vi "GrabImageDisplay.vi"(2 "error in (no error)":errorcluster, 3 "Image Src":T1, 4 "IBaseData":refnum<k24>) -> (0 "error out":errorcluster, 1 "Image out":T1)   [LabVIEW 2013, in "GxLVlib.lvlib"]
uses:
  GxLVlib.lvlib
  C:/Program Files/Daheng Imaging/GalaxySDK/Samples/LabVIEW SDK/x64/GxLVLib/dll/GxIAPINET.dll
  dll/GxIAPINET.dll
  <vilib>/vision/Image Controls.llb/IMAQ Image.ctl
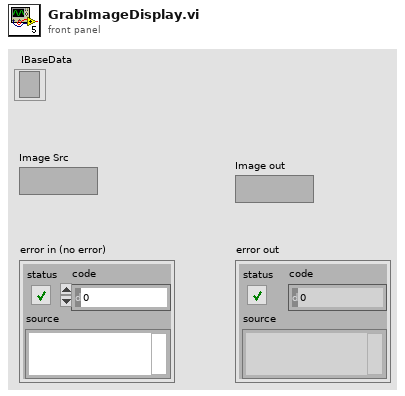
[diagram p1: front panel]
types:
  T1 = typedef "IMAQ Image.ctl" = refnum<image>
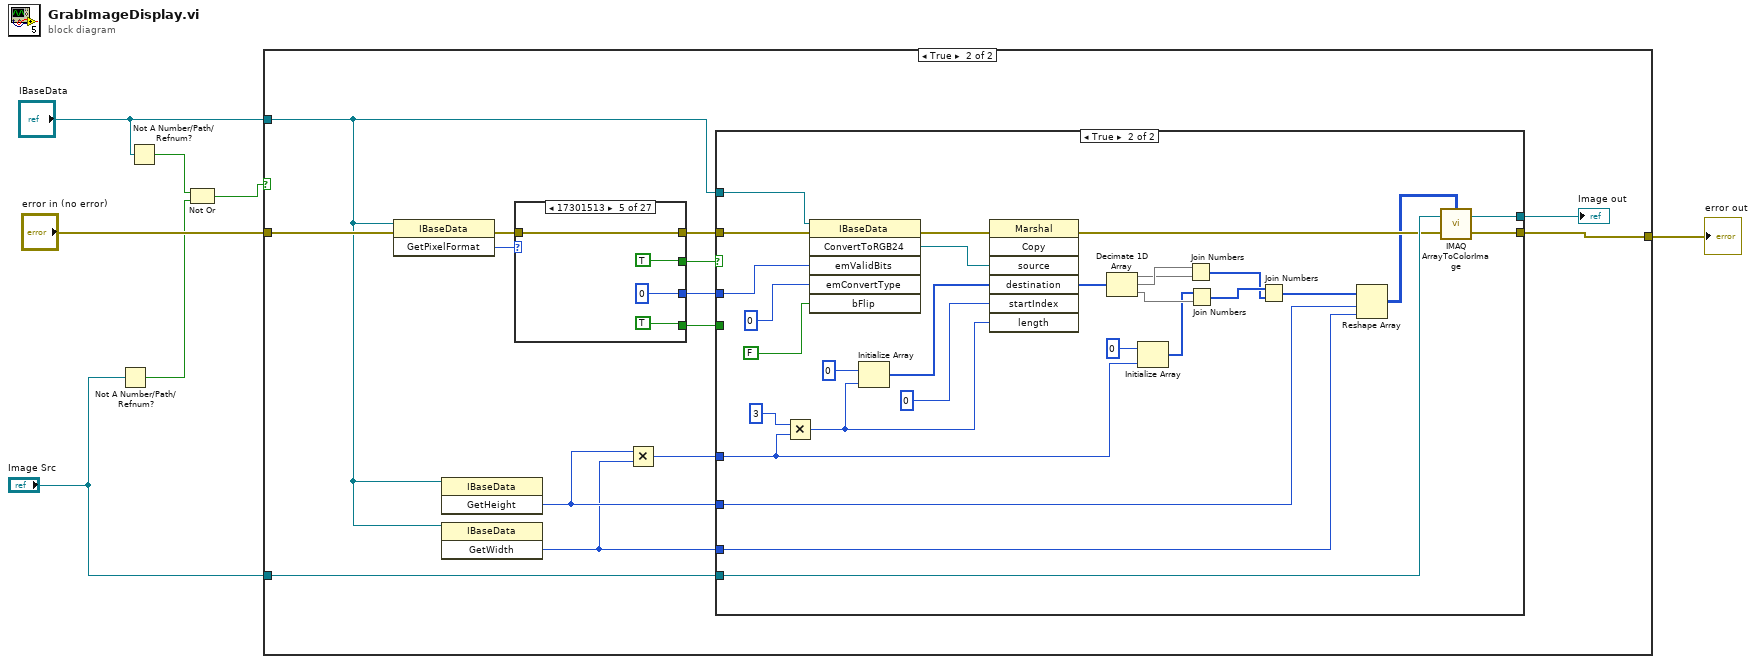
[diagram p0: block diagram]
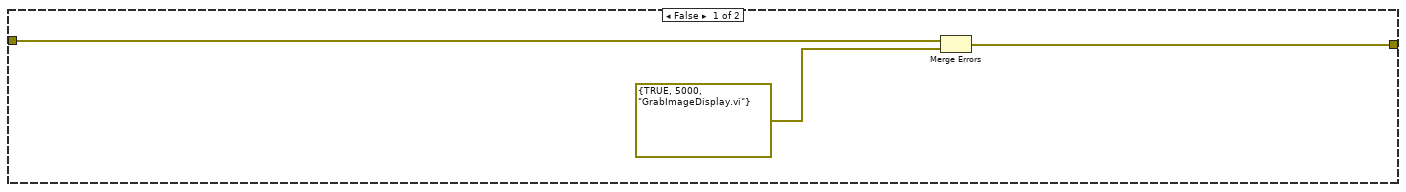
[diagram p2: hidden frame]
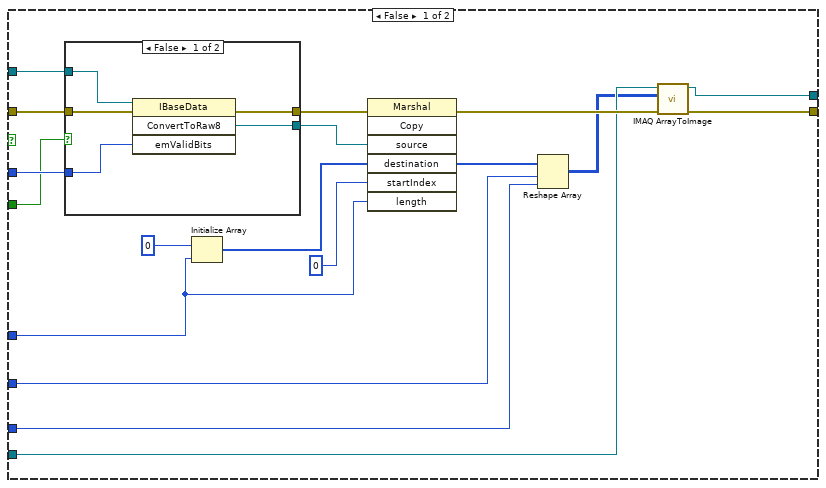
[diagram p3: hidden frame]
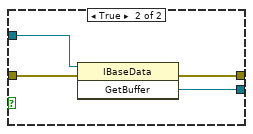
[diagram p4: hidden frame]
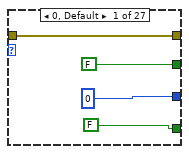
[diagram p5: hidden frame]
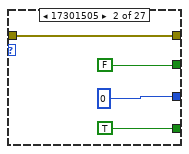
[diagram p6: hidden frame]
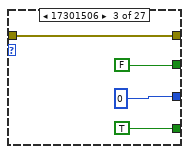
[diagram p7: hidden frame]
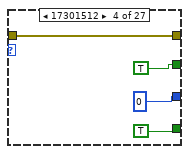
[diagram p8: hidden frame]
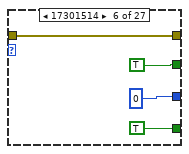
[diagram p9: hidden frame]
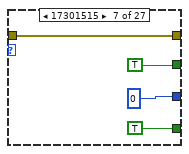
[diagram p10: hidden frame]
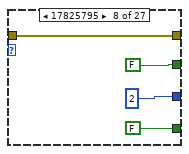
[diagram p11: hidden frame]
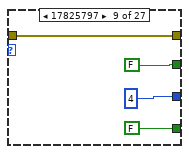
[diagram p12: hidden frame]
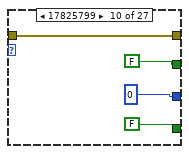
[diagram p13: hidden frame]
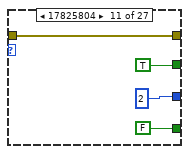
[diagram p14: hidden frame]
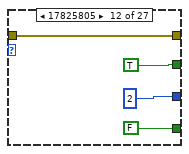
[diagram p15: hidden frame]
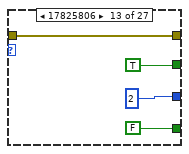
[diagram p16: hidden frame]
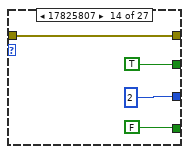
[diagram p17: hidden frame]
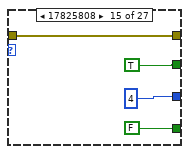
[diagram p18: hidden frame]
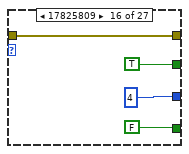
[diagram p19: hidden frame]
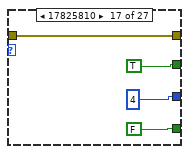
[diagram p20: hidden frame]
diagram:
  n1 = Not A Number/Path/Refnum?(number/path/refnum="Image Src") -> (NaN/Path/Refnum?=w3:bool)
  n2 = Not A Number/Path/Refnum?(number/path/refnum="IBaseData") -> (NaN/Path/Refnum?=w2:bool)
  n3 = Not Or(1:w3, 2:w2) -> (0:w1:bool)
  n4 = case shown="True" w1 {
    tunnel: "IBaseData" -> [_ w14]
    tunnel: "error in (no error)" -> [w10 w22]
    tunnel: [w8 w16] -> w5
    tunnel: "Image Src" -> [_ w17]
    frame False {
      n5 = Merge Errors(w10, errorcluster {TRUE, 5000, "GrabImageDisplay.vi"}) -> (w8:errorcluster)
    }
    frame True {
      n6 = invoke class="IBaseData" method="GetPixelFormat"(reference=w14, error in=w22) -> (error out=w19:errorcluster, "GetPixelFormat"=w21:i32)  [unwired: 1 in, 1 out]
      n7 = invoke class="IBaseData" method="GetHeight"(reference=w14) -> ("GetHeight"=w12:u64)  [unwired: 2 in, 2 out]
      n8 = invoke class="IBaseData" method="GetWidth"(reference=w14) -> ("GetWidth"=w11:u64)  [unwired: 2 in, 2 out]
      n9 = case shown="17301513" w21 {
        tunnel: [0 0 0 0 0 0 0 2 4 0 2 2 2 2 4 4 4 4 0 0 0 0 0 0 2 4 0] -> w23
        tunnel: [FALSE FALSE FALSE TRUE TRUE TRUE TRUE FALSE FALSE FALSE TRUE TRUE TRUE TRUE TRUE TRUE TRUE TRUE FALSE TRUE TRUE TRUE TRUE TRUE TRUE TRUE TRUE] -> w24
        tunnel: [FALSE TRUE TRUE TRUE TRUE TRUE TRUE FALSE FALSE FALSE FALSE FALSE FALSE FALSE FALSE FALSE FALSE FALSE FALSE FALSE FALSE FALSE FALSE FALSE FALSE FALSE FALSE] -> w20
        tunnel: w19 -> [w81 w85 w92 w96 w100 w104 w108 w112 w116 w120 w124 w128 w132 w136 w140 w144 w148 w152 w156 w160 w164 w168 w172 w176 w180 w184 w188]
        tunnel: [w81 w85 w92 w96 w100 w104 w108 w112 w116 w120 w124 w128 w132 w136 w140 w144 w148 w152 w156 w160 w164 w168 w172 w176 w180 w184 w188] -> w18
        frame 0, Default {
        }
        frame 17301505 {
        }
        frame 17301506 {
        }
        frame 17301512 {
        }
        frame 17301513 {
        }
        frame 17301514 {
        }
        frame 17301515 {
        }
        frame 17825795 {
        }
        frame 17825797 {
        }
        frame 17825799 {
        }
        frame 17825804 {
        }
        frame 17825805 {
        }
        frame 17825806 {
        }
        frame 17825807 {
        }
        frame 17825808 {
        }
        frame 17825809 {
        }
        frame 17825810 {
        }
        frame 17825811 {
        }
        frame 17825829 {
        }
        frame 17825838 {
        }
        frame 17825839 {
        }
        frame 17825840 {
        }
        frame 17825841 {
        }
        frame 35127329 {
        }
        frame 36700194 {
        }
        frame 36700195 {
        }
        frame 36700196 {
        }
      }
      n10 = Multiply(x=w12, y=w11) -> (x*y=w13:u64)
      n11 = case shown="True" w24 {
        tunnel: w23 -> [w42 w80]
        tunnel: w13 -> [w37 w58]
        tunnel: w20 -> [w35 _]
        tunnel: w14 -> [w36 w72]
        tunnel: w18 -> [w34 w71]
        tunnel: w17 -> [w31 w68]
        tunnel: [w29 w65] -> w16
        tunnel: [w25 w66] -> w15
        tunnel: w12 -> [w27 w64]
        tunnel: w11 -> [w26 w63]
        frame False {
          n12 = case shown="False" w35 {
            tunnel: w42 -> [w47 _]
            tunnel: [w46 w51] -> w41
            tunnel: w36 -> [w45 w50]
            tunnel: w34 -> [w44 w49]
            tunnel: [w43 w48] -> w33
            frame False {
              n13 = invoke class="IBaseData" method="ConvertToRaw8"(reference=w45, error in=w44, "emValidBits"=w47) -> (error out=w43:errorcluster, "ConvertToRaw8"=w46:refnum<k24>)  [unwired: 1 in, 2 out]
            }
            frame True {
              n14 = invoke class="IBaseData" method="GetBuffer"(reference=w50, error in=w49) -> (error out=w48:errorcluster, "GetBuffer"=w51:refnum<k24>)  [unwired: 1 in, 1 out]
            }
          }
          n15 = Initialize Array(u8 0, w37) -> (w40:u8[])
          n16 = invoke class="Marshal" method="Copy"(error in=w33, "source"=w41, "destination"=w40, "startIndex"=u8 0, "length"=w37) -> (error out=w32:errorcluster, "destination"=w28:u8[])  [unwired: 2 in, 5 out]
          n17 = Reshape Array(w28, w27, w26) -> (w30:u8[][])
          n18 = call "IMAQ ArrayToImage"("error in (no error)"=w32, "Image Pixels (U8)"=w30, "Image"=w31) -> ("error out"=w29:errorcluster, "Image Out"=w25:T1)  [unwired: 7 in]
        }
        frame True {
          n19 = Multiply(x=3, y=w58) -> (x*y=w70:u64)
          n20 = invoke class="IBaseData" method="ConvertToRGB24"(reference=w72, error in=w71, "emValidBits"=w80, "emConvertType"=0, "bFlip"=FALSE) -> (error out=w74:errorcluster, "ConvertToRGB24"=w77:refnum<k24>)  [unwired: 1 in, 4 out]
          n21 = Initialize Array(u8 0, w70) -> (w69:u8[])
          n22 = invoke class="Marshal" method="Copy"(error in=w74, "source"=w77, "destination"=w69, "startIndex"=u8 0, "length"=w70) -> (error out=w67:errorcluster, "destination"=w61:u8[])  [unwired: 2 in, 5 out]
          n23 = Decimate 1D Array(w61) -> (w56:u8[], w57:u8[], w55:u8[])
          n24 = Initialize Array(u8 0, w58) -> (w54:u8[])
          n25 = Join Numbers(hi=w57, lo=w56) -> ((hi.lo)=w52:u16[])
          n26 = Join Numbers(hi=w54, lo=w55) -> ((hi.lo)=w53:u16[])
          n27 = Join Numbers(hi=w53, lo=w52) -> ((hi.lo)=w60:u32[])
          n28 = Reshape Array(w60, w64, w63) -> (w62:u32[][])
          n29 = call "IMAQ ArrayToColorImage"("Image Pixels (U32)"=w62, "Image"=w68, "error in (no error)"=w67) -> ("Image Out"=w66:T1, "error out"=w65:errorcluster)  [unwired: 2 in]
        }
      }
      "Image out" <- w15
    }
  }
  "error out" <- w5
